vi "LCR_InsertMeasurements.vi"(4 "Data cluster":T1, 6 "TimeStamp":timestamp, 8 "error in (no error)":errorcluster, 9 "Data_IN":T4 {"GUI Data Cluster"."SBR" format="%08b"}, 10 "Cluster IN":T2={"General"={"Config.ini"=path "", "Default Logging Path"=path ""}, "Hardware"={"Global T VAR"="", "Global B VAR"="", "VISAS"={"GEN COM"="", "SCOPE COM"="", "VNA COM"=""}, "Connected?"={"SCOPE"=FALSE, "GEN"=FALSE, "VNA"=FALSE}}, "Operation"={"Operation Mode"=enum."Idle-Off", "Status"="", "NewLog?"=FALSE, "OvenWarn"=FALSE, "Scope Settings"={"TimeBase"=0.0, "VerticalScale"=4.0}}}) -> (0 "error out":errorcluster, 1 "Data_OUT":T4 {"GUI Data Cluster"."SBR" format="%08b"}, 2 "Cluster OUT":T2={"General"={"Config.ini"=path "", "Default Logging Path"=path ""}, "Hardware"={"Global T VAR"="", "Global B VAR"="", "VISAS"={"GEN COM"="", "SCOPE COM"="", "VNA COM"=""}, "Connected?"={"SCOPE"=FALSE, "GEN"=FALSE, "VNA"=FALSE}}, "Operation"={"Operation Mode"=enum."Idle-Off", "Status"="", "NewLog?"=FALSE, "OvenWarn"=FALSE, "Scope Settings"={"TimeBase"=0.0, "VerticalScale"=4.0}}})   [LabVIEW 2021]
uses:
  Data_Cluster.ctl
  Measurement_Cluster.ctl
  Config_Cluster.ctl
  Mode_Enum.ctl
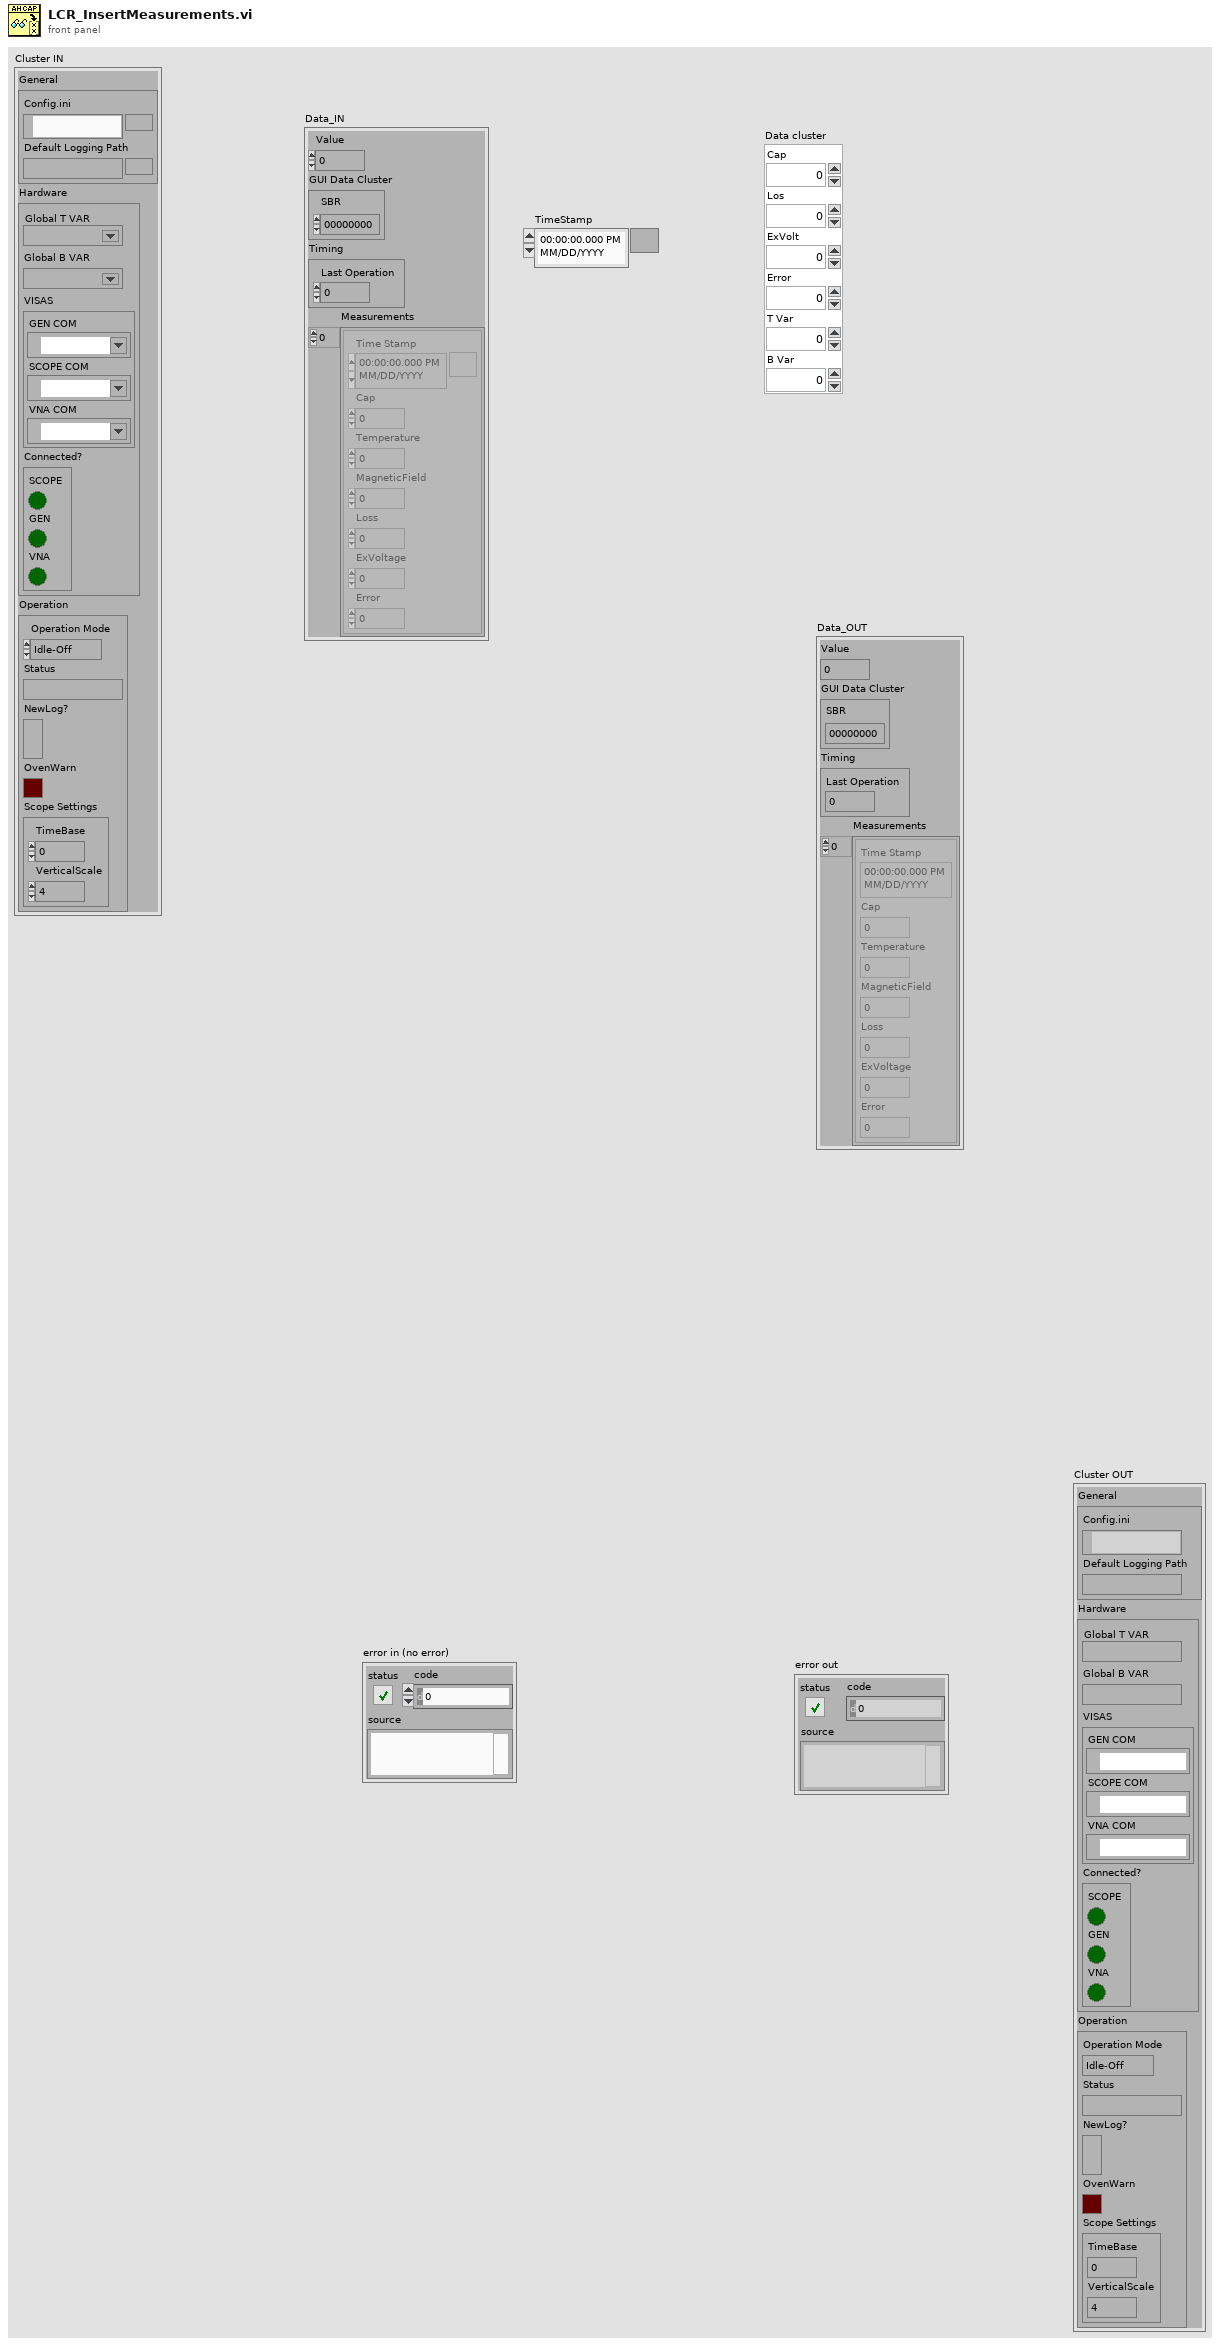
[diagram p1: front panel]
types:
  T1 = cluster{"Cap":dbl, "Los":dbl, "ExVolt":dbl, "Error":i32, "T Var":dbl, "B Var":dbl}
  T2 = typedef "Config_Cluster.ctl" = cluster{"General":cluster{"Config.ini":path, "Default Logging Path":path}, "Hardware":cluster{"Global T VAR":refnum<k21>, "Global B VAR":refnum<k21>, "VISAS":cluster{"GEN COM":refnum<visa-resource-name>, "SCOPE COM":refnum<visa-resource-name>, "VNA COM":refnum<visa-resource-name>}, "Connected?":cluster{"SCOPE":bool, "GEN":bool, "VNA":bool}}, "Operation":cluster{"Operation Mode":T3, "Status":string, "NewLog?":bool, "OvenWarn":bool, "Scope Settings":cluster{"TimeBase":dbl, "VerticalScale":dbl}}}
  T3 = typedef "Mode_Enum.ctl" = enum16{"Logging", "Idle-Off", "Idle"}
  T4 = typedef "Data_Cluster.ctl" = cluster{"Value":dbl, "GUI Data Cluster":cluster{"SBR":u16}, "Timing":cluster{"Last Operation":dbl}, "Measurements":T5[]}
  T5 = typedef "Measurement_Cluster.ctl" = cluster{"Time Stamp":timestamp, "Cap":dbl, "Temperature":dbl, "MagneticField":dbl, "Loss":dbl, "ExVoltage":dbl, "Error":dbl}
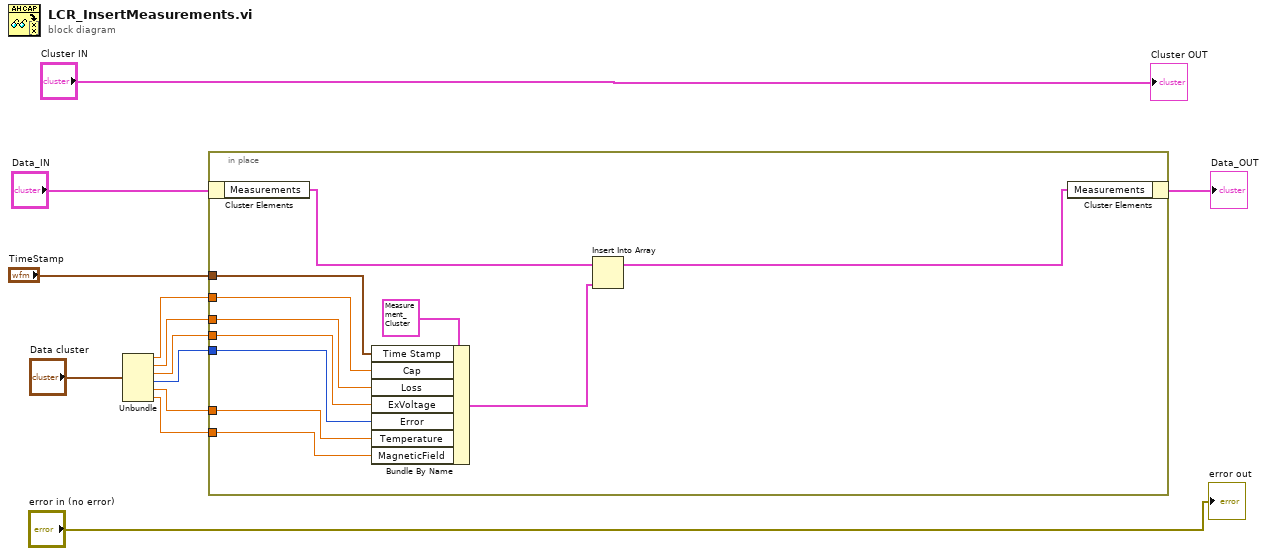
[diagram p0: block diagram]
diagram:
  n1 = Unbundle("Data cluster") -> ("Cap"=w9:dbl, "Los"=w5:dbl, "ExVolt"=w4:dbl, "Error"=w3:i32, "T Var"=w2:dbl, "B Var"=w1:dbl)
  n2 = in-place {
    in-place-border: "TimeStamp" -> [w21]
    in-place-border: w9 -> [w20]
    in-place-border: w5 -> [w19]
    in-place-border: w4 -> [w16]
    in-place-border: w3 -> [w15]
    in-place-border: w2 -> [w14]
    in-place-border: w1 -> [w13]
    n3 = in-place-cluster #1("Data_IN") -> ("Measurements"=w23:T5[])
    n4 = Bundle By Name(cluster=T5 {"Time Stamp"=timestamp(0 s since 1904-01-01), "Cap"=0.0, "Temperature"=0.0, "MagneticField"=0.0, "Loss"=0.0, "ExVoltage"=0.0, "Error"=0.0} ("new element/subarray"), "Time Stamp"=w21, "Cap"=w20, "Loss"=w19, "ExVoltage"=w16, "Error"=w15, "Temperature"=w14, "MagneticField"=w13) -> (w18:T5)
    n5 = Insert Into Array(array=w23, new element=w18) -> (w17:T5[])  [unwired: 1 in]
    n6 = in-place-cluster #1("Measurements"=w17) -> (→"Data_OUT":T4)
  }
  "Cluster OUT" <- "Cluster IN"
  "error out" <- "error in (no error)"
